vi "Set PNSN.vi"(8 "error in":errorcluster, 10 "Barcode":string="P:10-000001R:04S:QMC2200123", 11 "PreUUT in":refnum<class "PreUUT.lvclass">) -> (0 "error out":errorcluster, 2 "Found?":bool, 3 "PreUUT out":refnum<class "PreUUT.lvclass">)   [LabVIEW 2019, in "Sequence Main.lvlib" / "PreUUT.lvclass"]
uses:
  PreUUT.lvclass
  PreUUT.lvclass/PreUUT.ctl
  <vilib>/addons/TestStand/_TSUtility.llb/TestStand - Get Property Value (String).vi
  <vilib>/addons/TestStand/_TSUtility.llb/TestStand - Set Property Value (String).vi
  <vilib>/regexp/Match Regular Expression.xnode
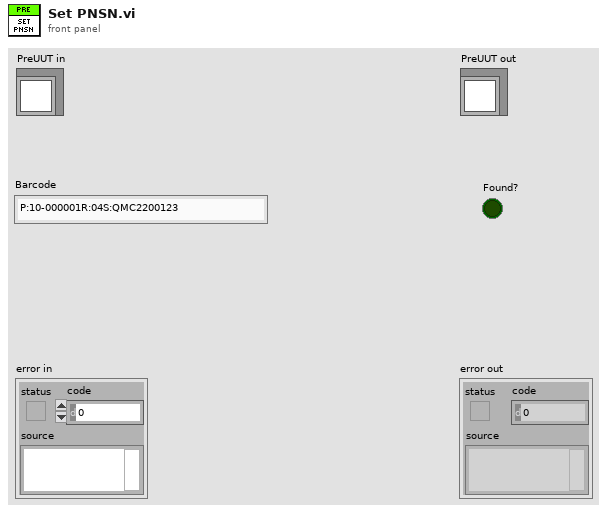
[diagram p1: front panel]
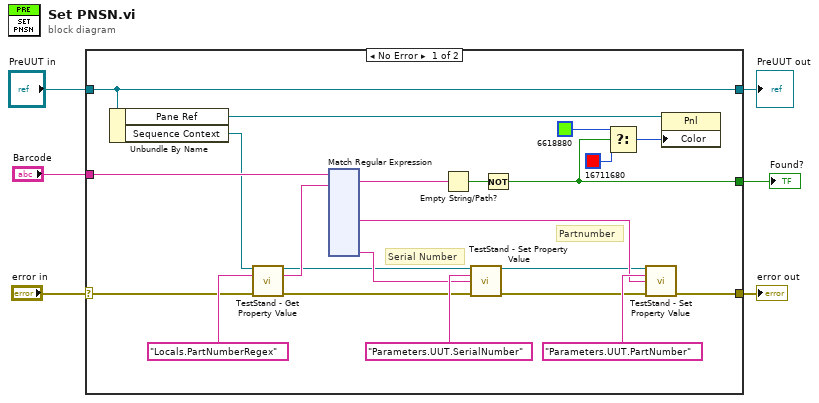
[diagram p0: block diagram]
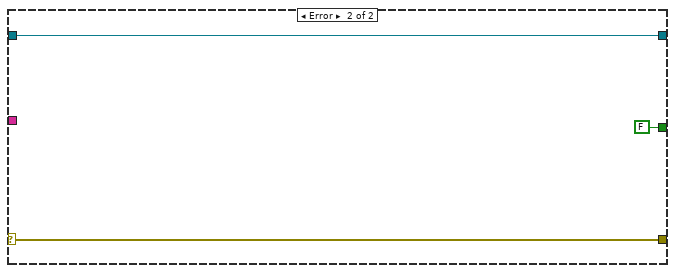
[diagram p2: hidden frame]
diagram:
  n1 = case shown="No Error" "error in" {
    selector: "error in" -> [w23 w152]
    tunnel: [w16 w152] -> w5
    tunnel: [w27 w151] -> w3
    tunnel: "PreUUT in" -> [w27 w151]
    tunnel: "Barcode" -> [w28 _]
    tunnel: [w10 FALSE] -> w1
    frame No Error {
      # "Serial Number"
      # "Partnumber"
      n2 = Unbundle By Name(w27) -> ("Pane Ref"=w11:refnum<vi>, "Sequence Context"=w26:refnum<k7>)
      n3 = call-poly <vilib>:"TestStand - Get Property Value.vi"("Sequence Context In"=w26, "Lookup String"="Locals.PartNumberRegex", "error in (no error)"=w23) -> ("Sequence Context Out"=w14:refnum<k7>, "Value"=w24:string, "error out"=w15:errorcluster)  [unwired: 10 in]
      n4 = xnode "Match Regular Expression"("input string"=w28, "regular expression"=w24) -> ("whole match"=w12:string, "submatch 2"=w18:string, "submatch 6"=w19:string)  [unwired: 4 in, 8 out]
      n5 = Empty String/Path?(string/path=w12) -> (empty?=w13:bool)
      n6 = call-poly <vilib>:"TestStand - Set Property Value.vi"("Sequence Context In"=w14, "Lookup String"="Parameters.UUT.SerialNumber", "New Value"=w19, "error in (no error)"=w15) -> ("Sequence Context Out"=w17:refnum<k7>, "error out"=w21:errorcluster)  [unwired: 10 in]
      n7 = Not(x=w13) -> (.not. x?=w10:bool)
      n8 = Select(t=u32 6618880 ("Color Box"), s=w10, f=u32 16711680 ("Color Box")) -> (s? t:f=w8:u32)
      n9 = call-poly <vilib>:"TestStand - Set Property Value.vi"("Sequence Context In"=w17, "Lookup String"="Parameters.UUT.PartNumber", "New Value"=w18, "error in (no error)"=w21) -> ("error out"=w16:errorcluster)  [unwired: 10 in, 1 out]
      n10 = property class="Pnl"(reference=w11, "Color"=w8) -> ()  [unwired: 1 in, 2 out]
    }
    frame Error {
    }
  }
  "error out" <- w5
  "PreUUT out" <- w3
  "Found?" <- w1
